vi "FEA_Model_Initialize_LEMP.vi"(11 "FEA_Model in":refnum<class "FEA_Model.lvclass">) -> (3 "FEA_Model out":refnum<class "FEA_Model.lvclass">)   [LabVIEW 2021, in "FEA_Model.lvclass"]
uses:
  FEA_Model.lvclass
  FEA_Model.lvclass/FEA_Model.ctl
  <vilib>/Analysis/Matrix/Numeric/Conversions/Matrix To Array - CM.vi
  <vilib>/Analysis/Matrix/NI_Matrix.lvlib
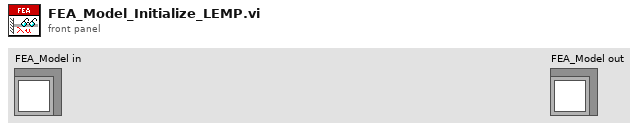
[diagram p1: front panel]
types:
  T1 = cluster{"Eigenvalues":dbl[], "Square Transpose Eigenvectors":dbl[][], "1/deltaStiff":dbl}
  T2 = enum16{"Particles to Nodes", "Particle to Node", "Nodes to Particles", "Node to Particle"}
  T3 = typedef "NI_Matrix.lvlib/ComplexMatrix.ctl" = cdb[][]
  T4 = enum16{"Scalar Particle to Meter", "Scalar Node to Meter", "Scalar Meter to Particle", "Scalar Meter to Node", "Array Particle to Meter", "Array Node to Meter", "Array Meter to Particle", "Array Meter to Node"}
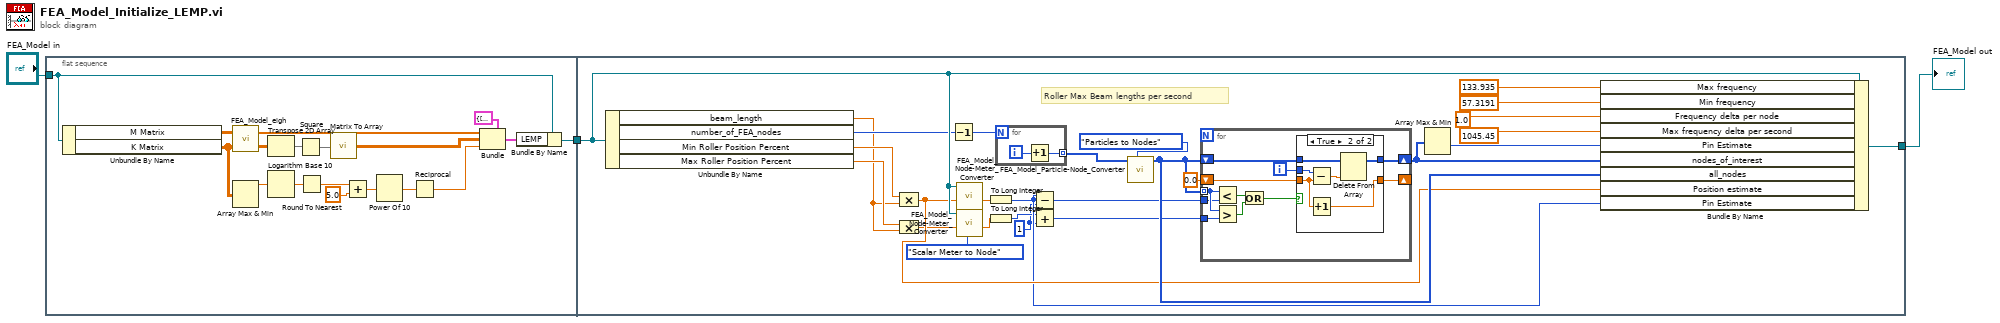
[diagram p0: block diagram]
diagram:
  n1 = flat-sequence {
    tunnel: "FEA_Model in" -> [w5]
    tunnel: [w4] -> w2
    tunnel: [w38] -> w1
    tunnel: w2 -> [w48]
    frame #0 {
      n2 = Unbundle By Name(w5) -> ("M Matrix"=w8:dbl[][], "K Matrix"=w7:dbl[][])
      n3 = call "FEA_Model_eigh.vi"("Stiffness"=w7, "Mass"=w8) -> ("Eigenvectors"=w13:T3, "Eigenvalues"=w11:dbl[])
      n4 = Array Max & Min(array=w7) -> (max value=w14:dbl)  [unwired: 3 out]
      n5 = Transpose 2D Array(2D array=w13) -> (transposed array=w21:T3)
      n6 = Logarithm Base 10(1:w14) -> (0:w17:dbl)
      n7 = Square(x=w21) -> (x^2=w20:T3)
      n8 = Round To Nearest(number=w17) -> (nearest integer value=w18:dbl)
      n9 = call-poly <vilib>:"Matrix To Array.vi"("Complex Matrix"=w20) -> ("Complex 2D Array"=w10:cdb[][])
      n10 = Add(x=w18, y=5.0) -> (x+y=w19:dbl)
      n11 = Power Of 10(x=w19) -> (10^x=w15:dbl)
      n12 = Reciprocal(x=w15) -> (1/x=w9:dbl)
      n13 = Bundle(cluster=T1 {"Eigenvalues"=[], "Square Transpose Eigenvectors"=[], "1/deltaStiff"=0.0} ("LEMP"), "Eigenvalues"=w11, "Square Transpose Eigenvectors"=w10, "1/deltaStiff"=w9) -> (w6:T1)
      n14 = Bundle By Name(cluster=w5, "LEMP"=w6) -> (w4:refnum<class "FEA_Model.lvclass">)
    }
    frame #1 {
      w25 = 1 ("y")
      w33 = T4."Scalar Meter to Node" ("Conversion Mode")
      # "Roller Max Beam lengths per second"
      n15 = Unbundle By Name(w48) -> ("beam_length"=w24:dbl, "number_of_FEA_nodes"=w37:i32, "Min Roller Position Percent"=w34:dbl, "Max Roller Position Percent"=w35:dbl)
      n16 = Compound Arithmetic op=MULTIPLY(w34, w24) -> (w40:dbl)
      n17 = Compound Arithmetic op=MULTIPLY(w35, w24) -> (w32:dbl)
      n18 = Decrement(x=w37) -> (x-1=w29:i32)
      n19 = call "FEA_Model_Node-Meter_Converter.vi"("Conversion Mode"=w33, "Scalar in"=w40, "FEA_Model in"=w48) -> ("Scalar out"=w31:dbl)  [unwired: 5 in, 3 out]
      n20 = call "FEA_Model_Node-Meter_Converter.vi"("Conversion Mode"=w33, "Scalar in"=w32, "FEA_Model in"=w48) -> ("Scalar out"=w30:dbl)  [unwired: 5 in, 3 out]
      n21 = To Long Integer(number=w31) -> (32bit integer=w39:i32)
      n22 = To Long Integer(number=w30) -> (32bit integer=w27:i32)
      n23 = for {
        N: w29 -> [_]
        tunnel: [w68] -> w23 mode=indexing
        i -> [w69]
        n24 = Increment(x=w69) -> (x+1=w68:i32)
      }
      n25 = Subtract(x=w39, y=w25) -> (x-y=w28:i32)
      n26 = Add(x=w27, y=w25) -> (x+y=w26:i32)
      n27 = call "FEA_Model_Particle-Node_Converter.vi"("mode"=T2."Particles to Nodes", "Particles"=w23) -> ("Nodes"=w41:i32[])  [unwired: 6 in, 3 out]
      n28 = for {
        tunnel: w41 -> [w52] mode=indexing
        shift-right: [w55] -> w42
        shift-left: w41 -> [w59]
        shift-right: [w54] -> _
        shift-left: 0.0 -> [w53]
        tunnel: w28 -> [w50]
        tunnel: w26 -> [w49]
        i -> [w51]
        n29 = Less?(x=w52, y=w50) -> (x < y?=w56:bool)
        n30 = Greater?(x=w52, y=w49) -> (0:w58:bool)
        n31 = Or(x=w56, y=w58) -> (x .or. y?=w57:bool)
        n32 = case shown="True" w57 {
          tunnel: w59 -> [w61 w66]
          tunnel: [w61 w67] -> w55
          tunnel: [w60 w65] -> w54
          tunnel: w53 -> [w60 w64]
          tunnel: w51 -> [_ w63]
          frame False {
          }
          frame True {
            n33 = Subtract(x=w63, y=w64) -> (x-y=w62:dbl)
            n34 = Increment(x=w64) -> (x+1=w65:dbl)
            n35 = Delete From Array(array=w66, index=w62) -> (array with subset deleted=w67:i32[])  [unwired: 1 in, 1 out]
          }
        }
      }
      n36 = Array Max & Min(array=w42) -> (min value=w43:i32)  [unwired: 3 out]
      n37 = Bundle By Name(cluster=w48, "Max frequency"=133.935, "Min frequency"=57.3191, "Frequency delta per node"=1.0, "Max frequency delta per second"=1045.45, "Pin Estimate"=w43, "nodes_of_interest"=w42, "all_nodes"=w41, "Position estimate"=w40, "Pin Estimate"=w39) -> (w38:refnum<class "FEA_Model.lvclass">)
    }
  }
  "FEA_Model out" <- w1
